vi "Control_DebounceDigital.vi"(0 "Input Signal":bool, 1 "Cycles to Filter":u16=5) -> (2 "Output Filtered Signal":bool)   [LabVIEW 2018]
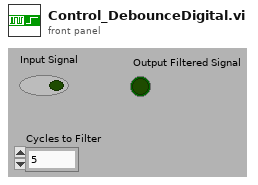
[diagram p1: front panel]
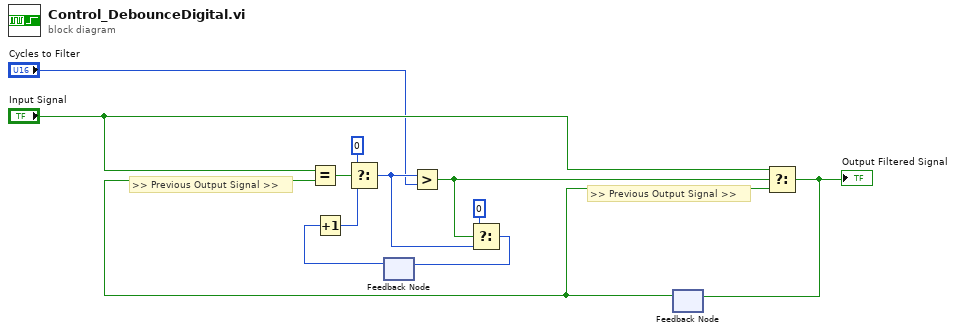
[diagram p0: block diagram]
diagram:
  # ">> Previous Output Signal >>"
  # ">> Previous Output Signal >>"
  n1 = feedback #1() -> (w11:u16)  [unwired: 1 out]
  n2 = Increment(x=w11) -> (x+1=w6:u16)
  n3 = feedback #2() -> (w8:bool)  [unwired: 1 out]
  n4 = Equal?(x="Input Signal", y=w8) -> (x = y?=w9:bool)
  n5 = Select(t=u16 0 ("f"), s=w9, f=w6) -> (s? t:f=w3:u16)
  n6 = Greater?(x=w3, y="Cycles to Filter") -> (0:w5:bool)
  n7 = Select(t=u16 0, s=w5, f=w3) -> (s? t:f=w4:u16)
  n8 = feedback-in #1(w4) -> ()
  n9 = Select(t="Input Signal", s=w5, f=w8) -> (s? t:f=w12:bool)
  "Output Filtered Signal" <- w12
  n10 = feedback-in #2(w12) -> ()
